vi "TRITON_SET_CLDN_COMMAND.vi"() -> (0 "Command String":string="p.pressures()")   [LabVIEW 2009]
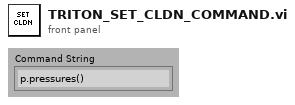
[diagram p1: front panel]
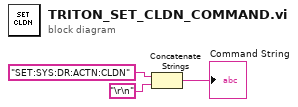
[diagram p0: block diagram]
diagram:
  n1 = Concatenate Strings("SET:SYS:DR:ACTN:CLDN", "\r\n") -> (→"Command String":string)
